vi "Ans_Step1.vi"   [LabVIEW 2012]
uses:
  <vilib>/NXT/Subs/MotorOutput.ctl
types:
  T1 = typedef "MotorOutput.ctl" = u8
  T2 = typedef "LVHSConnector.ctl" = refnum<class "BrickReference.lvclass">
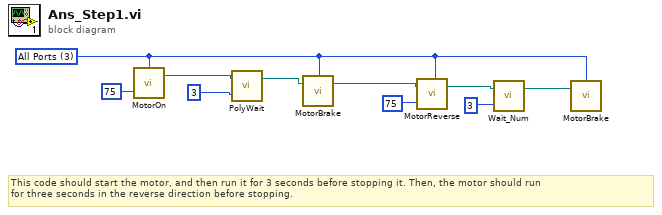
[diagram p0: block diagram]
diagram:
  w4 = T1 3 items=["Port A"=0, "Port B"=1, "Port C"=2, "Ports A & B"=4, "Ports A & C"=5, "Ports B & C"=6, "All Ports"=3] ("Output Port (All Ports)")
  # "This code should start the motor, and then run it for 3 seconds before stopping it. Then, the motor should run \nfor three seconds in the reverse direction before stopping."
  n1 = call <vilib>:"MotorOn.vi"("Power (75)"=75, "Output Port (All Ports)"=w4) -> ("NXT/EV3"=w10:T2)  [unwired: 2 in]
  n2 = call-poly <vilib>:"PolyWait.vi"("Time (1 sec)"=3, "NXT/EV3"=w10) -> ("NXT/EV3"=w8:T2)  [unwired: 2 in]
  n3 = call <vilib>:"MotorBrake.vi"("NXT/EV3"=w8, "Port (All Ports)"=w4) -> ("NXT/EV3"=w1:T2)  [unwired: 2 in]
  n4 = call <vilib>:"MotorReverse.vi"("Power (75)"=75, "NXT/EV3"=w1, "Output Port (All Ports)"=w4) -> ("NXT/EV3"=w6:T2)  [unwired: 1 in]
  n5 = call <vilib>:"Wait_Num.vi"("Time (1 sec)"=3, "NXT/EV3"=w6) -> ("NXT/EV3"=w5:T2)  [unwired: 2 in]
  n6 = call <vilib>:"MotorBrake.vi"("NXT/EV3"=w5, "Port (All Ports)"=w4) -> ()  [unwired: 2 in, 1 out]
